vi "Lanceur.vi"(9 "Shoot":bool, 10 "Accelerate":bool) -> ()   [LabVIEW 2019]
uses:
  <vilib>/Rock Robotics/WPI/ThirdParty/Phoenix-LabVIEW/Motor Controller/Controls/CTRE_Phoenix_MotorControl_FeedbackDevice.ctl
  <vilib>/Rock Robotics/WPI/ThirdParty/Phoenix-LabVIEW/Motor Controller/Controls/CTRE_Phoenix_MotorControl_ControlMode.ctl
  <vilib>/Rock Robotics/WPI/ThirdParty/Phoenix-LabVIEW/Motor Controller/Get/CTRE_Phoenix_MotorController_GetSupplyAndStatorCurrent_Enhanced.vi
  <vilib>/Rock Robotics/WPI/ThirdParty/Phoenix-LabVIEW/Motor Controller/Get/CTRE_Phoenix_MotorController_GetVoltage.vi
  <vilib>/Rock Robotics/WPI/ThirdParty/Phoenix-LabVIEW/Motor Controller/Get/CTRE_Phoenix_MotorController_GetSelectedSensorData.vi
  Robot Global Data.vi
panel:
  out "Waiting to shoot":bool
  in  "Acceptable deceleration to continue shooting":i64=100 step=5
  in  "Acceptable error on aim (in degrees)":dbl=0.8 format="%#_13g"
  out "Motor Current Plot":T1(graph)
  in  "lower limit":dbl=0.4 step=0.01 format="%#_13g"
  in  "upper limit":dbl=0.9 step=0.01 format="%#_13g"
  in  "Multiplier":dbl=0.00015 format="%#_8f"
  in  "PID Target":i64=29400 step=50
  in  "PID Zone":u64=4000 step=50
  out "SensorPosUnits":i32
  out "Motor output Plot":cluster{"Percent Output":dbl}(graph)
  out "Target Velocity Units per 100ms":i64
  out "Sensor Velocity Units Per 100ms":i32
  in  "I Zone":dbl
  in  "F 2":dbl=0.01569999999999998 step=0.0001
  in  "D 2":dbl=0.5 step=0.0001
  in  "I 2":dbl step=0.0001
  in  "P 2":dbl=0.05 step=0.0001
  out "Applied Output":dbl
  out "Speed Closed Loop Plots":T2(graph)
  # "PID /"
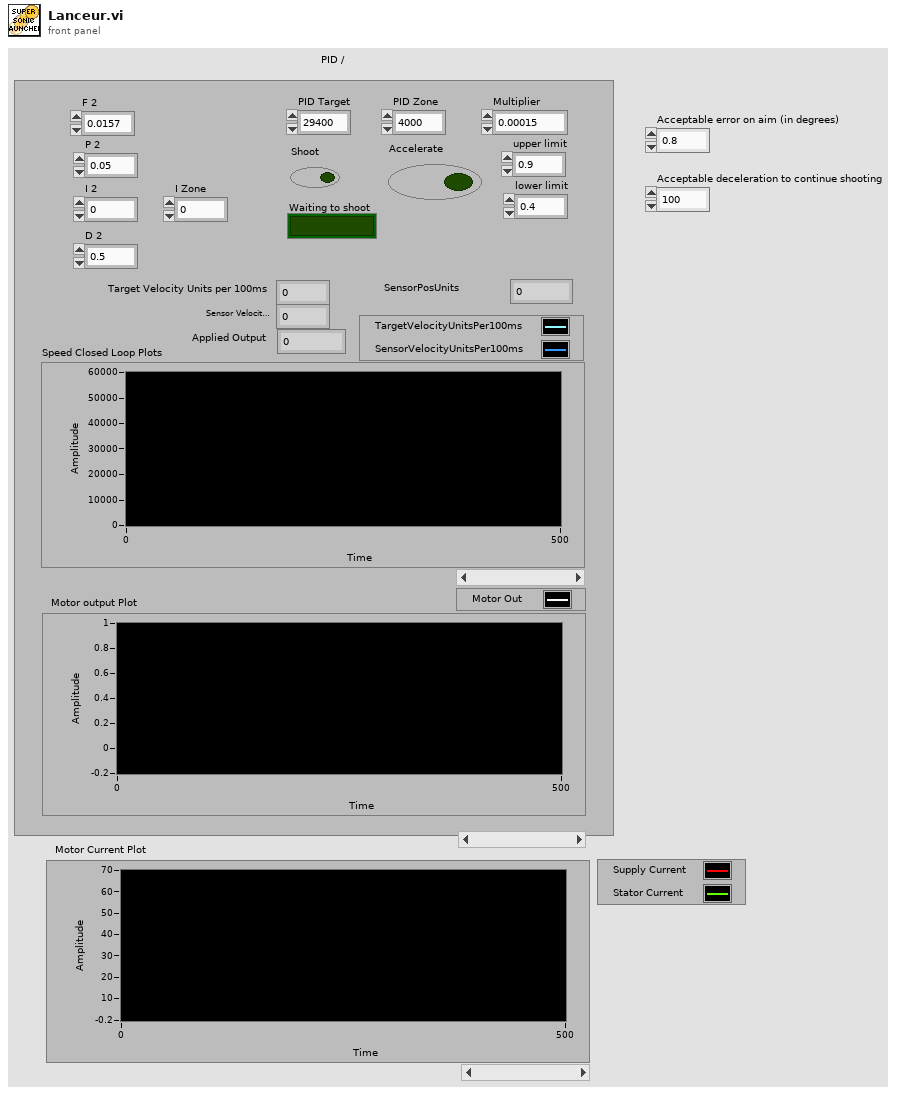
[diagram p1: front panel]
types:
  T1 = cluster{"Supply Current":dbl, "Stator Current":dbl}
  T2 = cluster{"x":dbl, "Velocity (Raw Sensor Units per 100 ms)":i32}
  T3 = typedef "CTRE_Phoenix_MotorControl_FeedbackDevice.ctl" = i8
  T4 = typedef "WPI_MotorControlDeviceRef.ctl" = cluster{"DeviceStatus":errorcluster, "Type":T5, "PWM":cluster{"PWM Channel":T6, "DeadBand":T7}, "CAN":cluster{"Device Number":u8, "SetOutput VI Ref":variant, "GetOutput VI Ref":variant, "Enable VI Ref":variant, "Disable VI Ref":variant, "Data":variant}, "Invert":bool, "DIO PWM":cluster{"PWM \"Enable\" Channel":T6, "DIOChannel":T8, "PWM Rate":dbl}}
  T5 = typedef "WPI_MotorControlType.ctl" = enum16{"PWM", "CAN", "DIO PWM"}
  T6 = typedef "FPGA_DIOPWMChannel.ctl" = enum8{"PWM 0", "PWM 1", "PWM 2", "PWM 3", "PWM 4", "PWM 5", "PWM 6", "PWM 7", "PWM 8", "PWM 9", "PWM MXP 0", "PWM MXP 1", "PWM MXP 2", "PWM MXP 3", "PWM MXP 4", "PWM MXP 5", "PWM MXP 6", "PWM MXP 7", "PWM MXP 8", "PWM MXP 9", "Invalid"}
  T7 = typedef "WPI_PWMDeadband.ctl" = cluster{"Name":string, "maxPositivePwm":i32, "minPositivePwm":i32, "centerPwm":i32, "maxNegativePwm":i32, "minNegativePwm":i32, "angularRange":u16}
  T8 = typedef "FPGA_DIOChannel.ctl" = enum8{"DIO 0", "DIO 1", "DIO 2", "DIO 3", "DIO 4", "DIO 5", "DIO 6", "DIO 7", "DIO 8", "DIO 9", "DIO MXP 0", "DIO MXP 1", "DIO MXP 2", "DIO MXP 3", "DIO MXP 4", "DIO MXP 5", "DIO MXP 6", "DIO MXP 7", "DIO MXP 8", "DIO MXP 9", "DIO MXP 10", "DIO MXP 11", "DIO MXP 12", "DIO MXP 13", "DIO MXP 14", "DIO MXP 15", "SPI Port CS1", "SPI Port CS2", "SPI Port CS3", "SPI Port MISO", "SPI Port MOSI", "Invalid"}
  T9 = typedef "CTRE_Phoenix_MotorControl_ControlMode.ctl" = u16
  T10 = cluster{"offsetAngle H":dbl, "offsetAngle V":dbl, "area":dbl, "skew":dbl, "target":dbl}
  T11 = cluster{"PID Target":dbl, "Velocity (Raw Sensor Units per 100 ms)":i32}
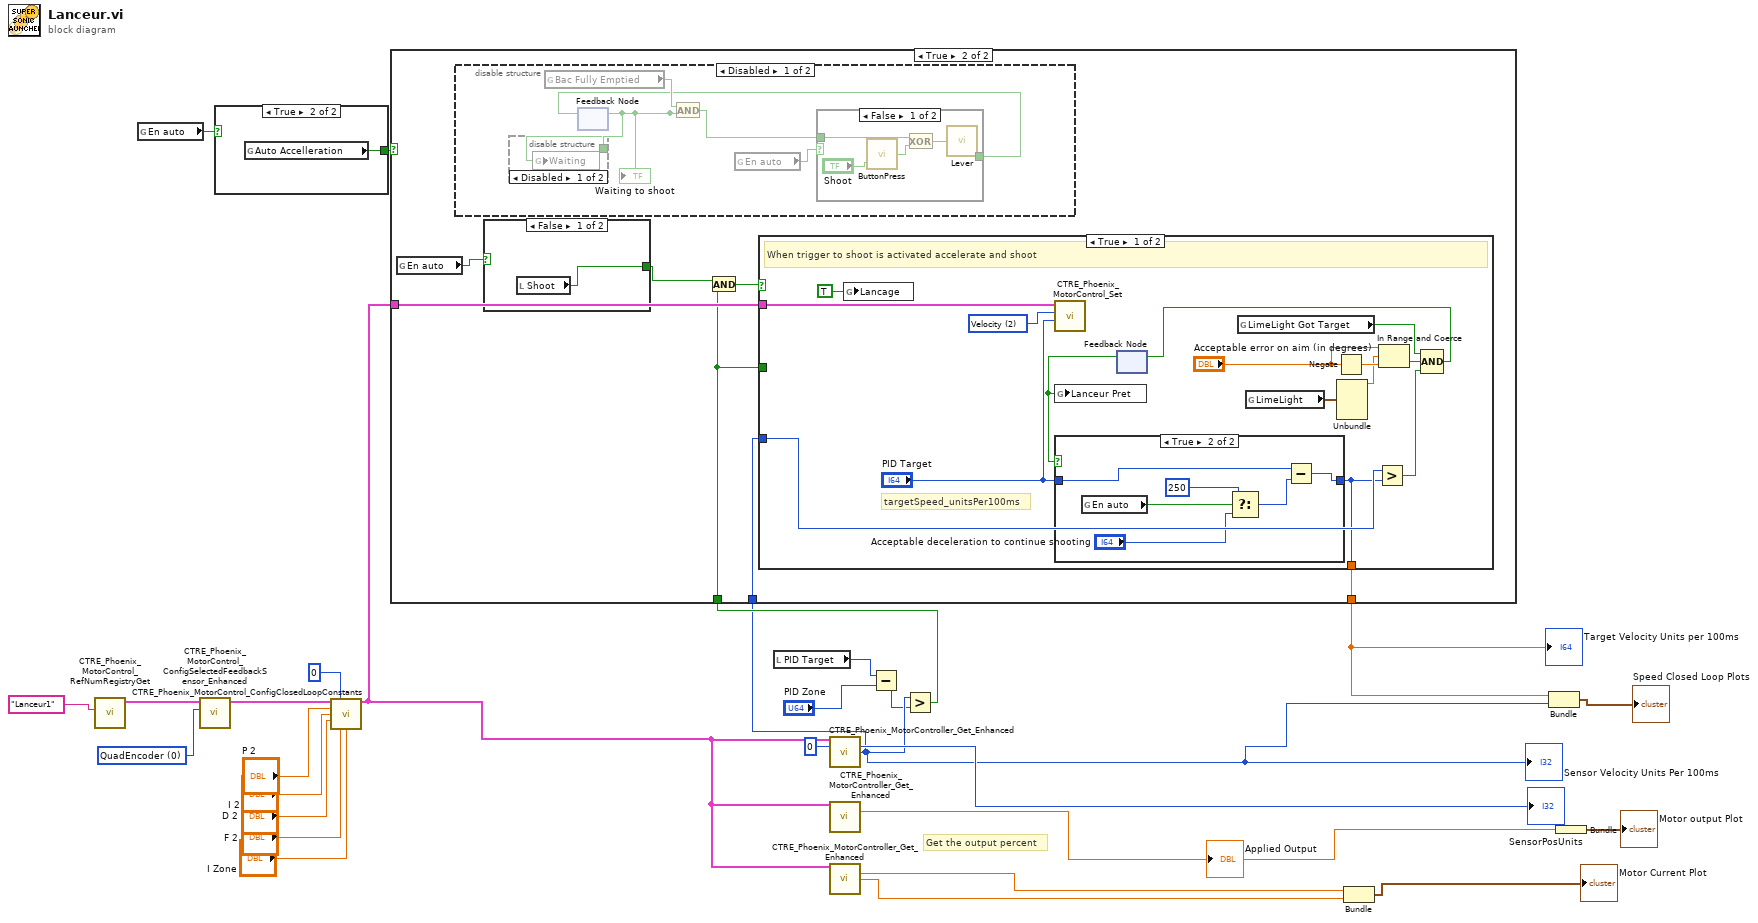
[diagram p0: block diagram]
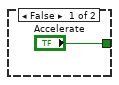
[diagram p2: hidden frame]
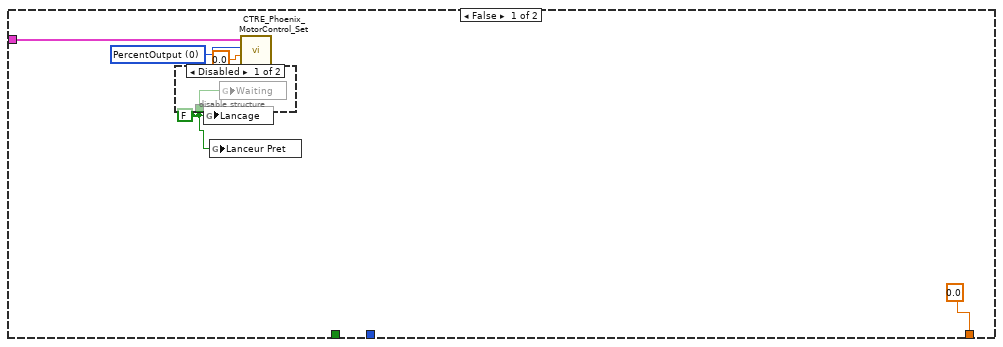
[diagram p3: hidden frame]
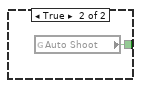
[diagram p6: hidden frame]
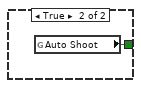
[diagram p8: hidden frame]
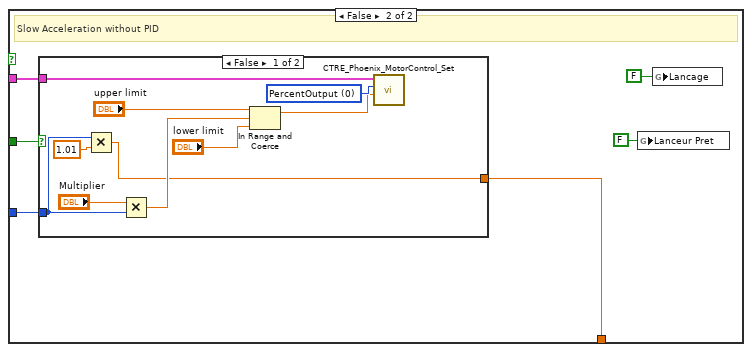
[diagram p10: hidden frame]
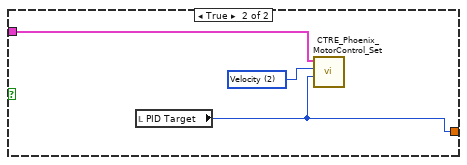
[diagram p11: hidden frame]
diagram:
  w16 = T3 0 items=["None"=-1, "QuadEncoder"=0, "Analog"=2, "Tachometer"=4, "Pulse Width Encoded Position"=8, "Sensor Sum (S0 + S1)"=9, "Sensor Difference (D0 - D1)"=10, "Remote Source 0"=11, "Remote Source 1"=12, "Software Emulated"=15] ("Feedback Device")
  # "Get the output percent"
  n1 = call <vilib>:"CTRE_Phoenix_MotorControl_RefNumRegistryGet.vi"("refnum name"="Lanceur1") -> ("PhoenixMotorControlDevRef"=w26:T4)  [unwired: 9 in, 1 out]
  n2 = global read "Robot Global Data.vi" "En auto"() -> (w2:bool)
  n3 = call <vilib>:"CTRE_Phoenix_MotorControl_ConfigSelectedFeedbackSensor_Enhanced.vi"("Feedback Device"=w16, "PhoenixMotorControlDevRef"=w26) -> ("PhoenixMotorControlDevRef"=w27:T4)  [unwired: 8 in, 1 out]
  n4 = case shown="True" w2 {
    tunnel: ["Accelerate" w29] -> w1
    frame False {
    }
    frame True {
      n5 = global read "Robot Global Data.vi" "Auto Accelleration"() -> (w29:bool)
    }
  }
  n6 = call <vilib>:"CTRE_Phoenix_MotorControl_ConfigClosedLoopConstants.vi"("PhoenixMotorControlDevRef"=w27, "slotIdx"=0, "P"="P 2", "I"="I 2", "D"="D 2", "F"="F 2", "I Zone"="I Zone") -> ("PhoenixMotorControlDevRef"=w12:T4)  [unwired: 7 in, 1 out]
  n7 = local read "PID Target"() -> (w6:i64)
  n8 = call-poly <vilib>:"CTRE_Phoenix_MotorController_Get_Enhanced.vi"("PhoenixMotorControlDevRef"=w12, "pidLoopIdx"=u32 0) -> ("Position (Raw Sensor Units)"=→"SensorPosUnits":i32, "Velocity (Raw Sensor Units per 100 ms)"=w14:i32)  [unwired: 10 in, 2 out]
  "Sensor Velocity Units Per 100ms" <- w14
  n9 = call-poly <vilib>:"CTRE_Phoenix_MotorController_Get_Enhanced.vi"("PhoenixMotorControlDevRef"=w12) -> ("Percent Output"=w19:dbl)  [unwired: 10 in, 4 out]
  "Applied Output" <- w19
  n10 = call-poly <vilib>:"CTRE_Phoenix_MotorController_Get_Enhanced.vi"("PhoenixMotorControlDevRef"=w12) -> ("Supply Current"=w10:dbl, "Stator Current"=w9:dbl)  [unwired: 11 in, 2 out]
  n11 = Subtract(x=w6, y="PID Zone") -> (x-y=w4:u64)
  n12 = Greater?(x=w14, y=w4) -> (0:w15:bool)
  n13 = case shown="True" w1 {
    tunnel: w12 -> [w33 w42]
    tunnel: w15 -> [_ w39]
    tunnel: w14 -> [_ w41]
    tunnel: [0.0 ("Speed For PID") w40] -> w8
    frame False {
      w30 = FALSE ("Enable Vision")
      w34 = T9 0 items=["PercentOutput"=0, "Position"=1, "Velocity"=2, "Current"=3, "Follower"=5, "MotionProfile"=6, "MotionMagic"=7, "MotionProfileArc"=10, "Disabled"=15] ("Control Mode")
      n14 = disable-structure shown="Disabled" {
        disable-tunnel: w30 -> [w35 _]
        frame Disabled {
          n15 = global write "Robot Global Data.vi" "Waiting"(w35) -> ()
        }
        frame Enabled {
        }
      }
      n16 = global write "Robot Global Data.vi" "Lancage"(w30) -> ()
      n17 = global write "Robot Global Data.vi" "Lanceur Pret"(w30) -> ()
      n18 = call <vilib>:"CTRE_Phoenix_MotorControl_Set.vi"("Output"=0.0, "Control Mode"=w34, "PhoenixMotorControlDevRef"=w33) -> ()  [unwired: 7 in, 2 out]
    }
    frame True {
      n19 = global read "Robot Global Data.vi" "En auto"() -> (w37:bool)
      n20 = disable-structure shown="Disabled" {
        frame Disabled {
          n21 = global read "Robot Global Data.vi" "Bac Fully Emptied"() -> (w47:bool)
          n22 = feedback #1() -> (w43:bool)  [unwired: 1 in]
          "Waiting to shoot" <- w43
          n23 = disable-structure shown="Disabled" {
            disable-tunnel: w43 -> [w48 _]
            frame Disabled {
              n24 = global write "Robot Global Data.vi" "Waiting"(w48) -> ()
            }
            frame Enabled {
            }
          }
          n25 = And(x=w47, y=w43) -> (x .and. y?=w44:bool)
          n26 = global read "Robot Global Data.vi" "En auto"() -> (w46:bool)
          n27 = case shown="False" w46 {
            tunnel: [w49 w54] -> w45
            tunnel: w44 -> [w50 _]
            frame False {
              n28 = call "ButtonPress.vi"("Input"="Shoot") -> ("Output"=w53:bool)  [unwired: 1 in]
              n29 = Exclusive Or(1:w53, 2:w50) -> (0:w51:bool)
              n30 = call "Lever.vi"("Input"=w51) -> ("Output"=w49:bool)
            }
            frame True {
              n31 = global read "Robot Global Data.vi" "Auto Shoot"() -> (w54:bool)
            }
          }
          n32 = feedback-in #1(w45) -> ()
        }
        frame Enabled {
        }
      }
      n33 = case shown="False" w37 {
        tunnel: [w55 w56] -> w36
        frame False {
          n34 = local read "Shoot"() -> (w55:bool)
        }
        frame True {
          n35 = global read "Robot Global Data.vi" "Auto Shoot"() -> (w56:bool)
        }
      }
      n36 = And(x=w36, y=w39) -> (x .and. y?=w38:bool)
      n37 = case shown="True" w38 {
        tunnel: w42 -> [w71 w84]
        tunnel: w41 -> [w67 w83]
        tunnel: [w62 w82] -> w40
        tunnel: w39 -> [_ w79]
        frame True {
          w70 = T9 2 items=["PercentOutput"=0, "Position"=1, "Velocity"=2, "Follower"=5, "MotionProfile"=6, "MotionMagic"=7, "MotionMagicArc"=8, "TimedPercentOutput"=9, "Disabled"=15] ("Control Mode")
          # "targetSpeed_unitsPer100ms"
          # "When trigger to shoot is activated accelerate and shoot"
          n38 = global write "Robot Global Data.vi" "Lancage"(TRUE ("Enable Vision")) -> ()
          n39 = call <vilib>:"CTRE_Phoenix_MotorControl_Set.vi"("Output"="PID Target", "Control Mode"=w70, "PhoenixMotorControlDevRef"=w71) -> ()  [unwired: 7 in, 2 out]
          n40 = feedback #2() -> (w63:bool)  [unwired: 1 in]
          n41 = global write "Robot Global Data.vi" "Lanceur Pret"(w63) -> ()
          n42 = case shown="True" w63 {
            tunnel: [w72 w77] -> w62
            tunnel: "PID Target" -> [w72 w78]
            frame False {
            }
            frame True {
              n43 = global read "Robot Global Data.vi" "En auto"() -> (w76:bool)
              n44 = Select(t=i64 250, s=w76, f="Acceptable deceleration to continue shooting") -> (s? t:f=w74:i64)
              n45 = Subtract(x=w78, y=w74) -> (x-y=w77:i64)
            }
          }
          n46 = global read "Robot Global Data.vi" "LimeLight Got Target"() -> (w57:bool)
          n47 = global read "Robot Global Data.vi" "LimeLight"() -> (w68:T10)
          n48 = Negate(x="Acceptable error on aim (in degrees)") -> (-x=w66:dbl)
          n49 = Unbundle(w68) -> ("offsetAngle H"=w59:dbl)  [unwired: 4 out]
          n50 = Greater?(x=w67, y=w62) -> (0:w61:bool)
          n51 = In Range and Coerce(upper limit="Acceptable error on aim (in degrees)", x=w59, lower limit=w66) -> (In Range?=w60:bool)  [unwired: 1 out]
          n52 = Compound Arithmetic op=AND(w57, w60, w61) -> (w58:bool)
          n53 = feedback-in #2(w58) -> ()
        }
        frame False {
          # "Slow Acceleration without PID"
          n54 = case shown="False" w79 {
            tunnel: w84 -> [w94 w96]
            tunnel: w83 -> [w93 _]
            tunnel: [w86 w95] -> w82
            frame False {
              w92 = T9 0 items=["PercentOutput"=0, "Position"=1, "Velocity"=2, "Current"=3, "Follower"=5, "MotionProfile"=6, "MotionMagic"=7, "MotionProfileArc"=10, "Disabled"=15] ("Control Mode")
              n55 = Multiply(x=w93, y=1.01) -> (x*y=w86:dbl)
              n56 = Multiply(x="Multiplier", y=w93) -> (x*y=w90:dbl)
              n57 = In Range and Coerce(upper limit="upper limit", x=w90, lower limit="lower limit") -> (coerced(x)=w85:dbl)  [unwired: 1 out]
              n58 = call <vilib>:"CTRE_Phoenix_MotorControl_Set.vi"("Output"=w85, "Control Mode"=w92, "PhoenixMotorControlDevRef"=w94) -> ()  [unwired: 7 in, 2 out]
            }
            frame True {
              w97 = T9 2 items=["PercentOutput"=0, "Position"=1, "Velocity"=2, "Follower"=5, "MotionProfile"=6, "MotionMagic"=7, "MotionMagicArc"=8, "TimedPercentOutput"=9, "Disabled"=15] ("Control Mode")
              n59 = local read "PID Target"() -> (w95:i64)
              n60 = call <vilib>:"CTRE_Phoenix_MotorControl_Set.vi"("Output"=w95, "Control Mode"=w97, "PhoenixMotorControlDevRef"=w96) -> ()  [unwired: 7 in, 2 out]
            }
          }
          n61 = global write "Robot Global Data.vi" "Lanceur Pret"(FALSE ("Lanceur Pret")) -> ()
          n62 = global write "Robot Global Data.vi" "Lancage"(FALSE ("Enable Vision")) -> ()
        }
      }
    }
  }
  "Target Velocity Units per 100ms" <- w8
  n63 = Bundle("Supply Current"=w10, "Stator Current"=w9) -> (→"Motor Current Plot":T1)  [unwired: 1 in]
  n64 = Bundle("PID Target"=w8, "Velocity (Raw Sensor Units per 100 ms)"=w14) -> (→"Speed Closed Loop Plots":T11)  [unwired: 1 in]
  n65 = Bundle("Percent Output"=w19) -> (→"Motor output Plot":cluster{"Percent Output":dbl})  [unwired: 1 in]
